vi "Read CS++Factory.vi"(8 "Error In":errorcluster, 11 "CS++RTMainActor in":refnum<class "CS++RTMainActor.lvclass">) -> (0 "Error Out":errorcluster, 2 "CS++Factory":refnum<class "CS++Factory.lvclass">, 3 "CS++RTMainActor out":refnum<class "CS++RTMainActor.lvclass">)   [LabVIEW 2015, in "CS++RTMain.lvlib" / "CS++RTMainActor.lvclass"]
doc: "Read Factory from attribute."
uses:
  CS++RTMainActor.lvclass
  CSPP_Core/Classes/CS++BaseClasses/Factory/CS++Factory.lvclass
  CS++RTMainActor.lvclass/CS++RTMainActor.ctl
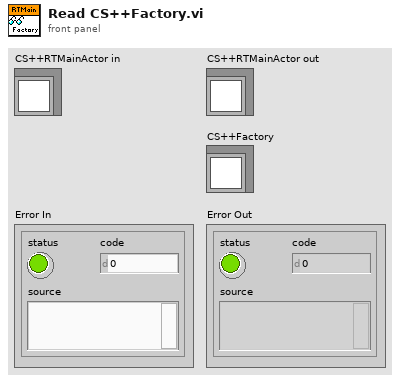
[diagram p1: front panel]
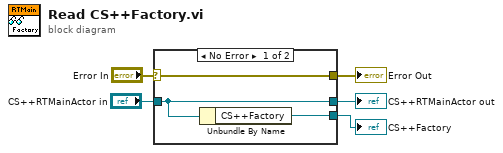
[diagram p0: block diagram]
diagram:
  n1 = case shown="No Error" "Error In" {
    selector: "Error In" -> [w8 w9]
    tunnel: [w8 w9] -> w4
    tunnel: [w7 w10] -> w2
    tunnel: "CS++RTMainActor in" -> [w7 w10]
    tunnel: [w6 _] -> w1
    frame No Error {
      n2 = Unbundle By Name(w7) -> ("CS++Factory"=w6:refnum<class "CS++Factory.lvclass">)
    }
    frame Error {
    }
  }
  "Error Out" <- w4
  "CS++RTMainActor out" <- w2
  "CS++Factory" <- w1
